vi "UpdateActualDepsOfLibraries.vi"(8 "error in (no error)":errorcluster, 9 "Status Indicator Ref":refnum<vi>, 10 "Lvlib paths":path[](array[path]), 11 "CLI in":refnum<class "CLI.lvclass">) -> (0 "error out":errorcluster, 3 "CLI out":refnum<class "CLI.lvclass">)   [LabVIEW 2023, in "DepsWatch.lvlib"]
uses:
  DepsWatch.lvlib
  <vilib>/Wiresmith Technology/G CLI/CLI Class/CLI.lvclass
  <vilib>/Utility/config.llb/NI_LVConfig.lvlib
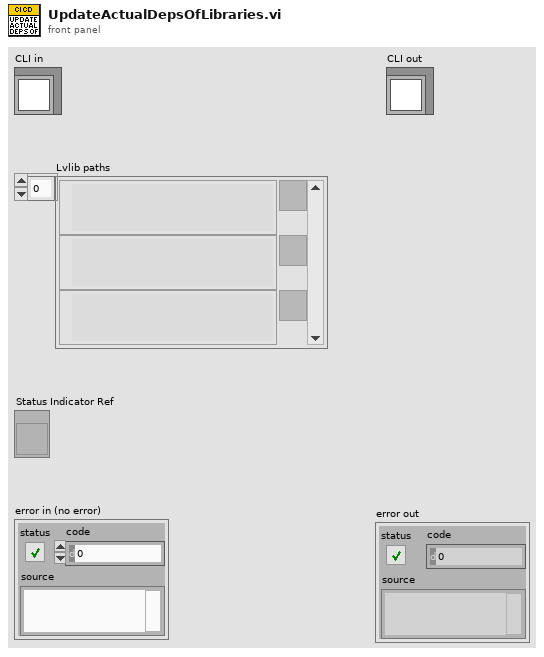
[diagram p1: front panel]
types:
  T1 = typedef "NI_LVConfig.lvlib/Config Data RefNum.ctl" = refnum<k1>
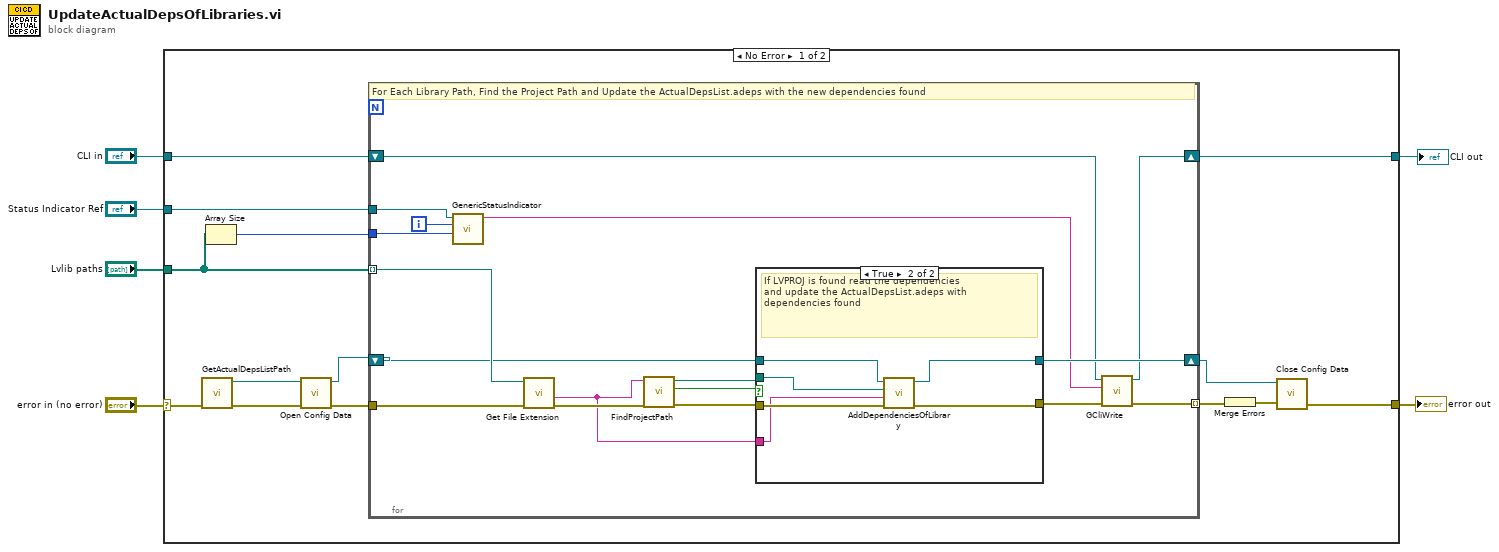
[diagram p0: block diagram]
diagram:
  n1 = case shown="No Error" "error in (no error)" {
    selector: "error in (no error)" -> [w8 w47]
    tunnel: "Status Indicator Ref" -> [w20 _]
    tunnel: [w19 w47] -> w5
    tunnel: [w18 w46] -> w4
    tunnel: "CLI in" -> [w17 w46]
    tunnel: "Lvlib paths" -> [w12 _]
    frame No Error {
      n2 = call "GetActualDepsListPath.vi"("error in (no error)"=w8) -> ("error out"=w16:errorcluster, "ActualDepsListPath"=w15:path)  [unwired: 9 in]
      n3 = Array Size(array=w12) -> (size(s)=w13:i32)
      n4 = call <vilib>:"Open Config Data.vi"("error in (no error)"=w16, "configuration file path"=w15) -> ("error out"=w7:errorcluster, "refnum"=w14:T1)  [unwired: 7 in, 1 out]
      n5 = for {
        tunnel: w7 -> [w37]
        tunnel: w12 -> [w36] mode=indexing
        tunnel: [w25] -> w9 mode=indexing
        shift-right: [w30] -> w11
        shift-left: w14 -> [w31]
        tunnel: w13 -> [w29]
        shift-right: [w24] -> w18
        shift-left: w17 -> [w22]
        tunnel: w20 -> [w27]
        i -> [w28]
        # "For Each Library Path, Find the Project Path and Update the ActualDepsList.adeps with the new dependencies found"
        n6 = call "GenericStatusIndicator.vi"("Total"=w29, "Current Iteration"=w28, "Status Indicator Ref In"=w27) -> ("CLI Status to Print"=w23:string)  [unwired: 8 in]
        n7 = call <vilib>:"Get File Extension.vi"("error in (no error)"=w37, "file"=w36) -> ("error out"=w35:errorcluster, "filename without extension"=w21:string)  [unwired: 5 in, 3 out]
        n8 = call "FindProjectPath.vi"("error in (no error)"=w35, "Library Name"=w21) -> ("error out"=w33:errorcluster, "Found?"=w34:bool, "Project Path"=w32:path)  [unwired: 7 in]
        n9 = case shown="True" w34 {
          tunnel: w33 -> [w39 w44]
          tunnel: [w39 w43] -> w26
          tunnel: w32 -> [_ w45]
          tunnel: w31 -> [w38 w42]
          tunnel: [w38 w41] -> w30
          tunnel: w21 -> [_ w40]
          frame False {
            # "If the Project path is not found ignore updating the ActualDepsList.adeps"
          }
          frame True {
            # "If LVPROJ is found read the dependencies \nand update the ActualDepsList.adeps with dependencies found"
            n10 = call "AddDependenciesOfLibrary.vi"("error in (no error)"=w44, "LibraryName"=w40, "Project Path"=w45, "Config Refnum in"=w42) -> ("error out"=w43:errorcluster, "Config Refnum out"=w41:T1)  [unwired: 5 in, 1 out]
          }
        }
        n11 = call "GCliWrite.vi"("error in (no error)"=w26, "Text to Write"=w23, "CLI in"=w22) -> ("error out"=w25:errorcluster, "CLI out"=w24:refnum<class "CLI.lvclass">)  [unwired: 7 in]
      }
      n12 = Merge Errors(w9) -> (w10:errorcluster)
      n13 = call <vilib>:"Close Config Data.vi"("error in (no error)"=w10, "refnum"=w11) -> ("error out"=w19:errorcluster)  [unwired: 8 in, 1 out]
    }
    frame Error {
    }
  }
  "error out" <- w5
  "CLI out" <- w4
